vi "Get Motor Temperature Config.vi"(7 "timeout (1s)":dbl=1.0 min=0.0, 8 "error in (no error)":errorcluster, 11 "SDO object in":refnum<k20>) -> (0 "error out":errorcluster, 1 "completion codes":u32[](array[numeric]), 3 "SDO object out":refnum<k20>, 4 "Motor Temperature Config":T1)   [LabVIEW 2016]
uses:
  <vilib>/CANopenLib/CANOPEN.llb/CANopen SDO Read [U8].vi
  <vilib>/CANopenLib/CANOPEN.llb/CANopen SDO Read [I16].vi
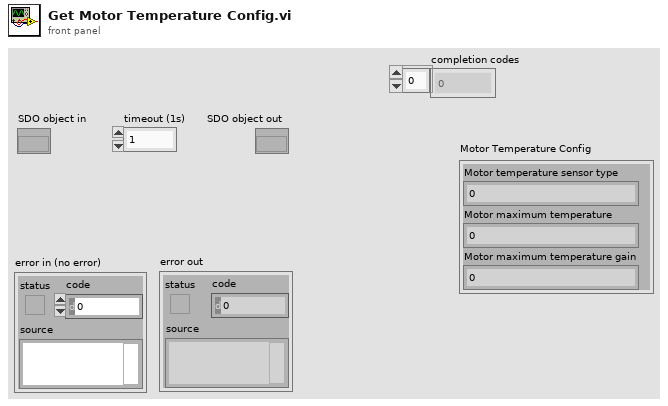
[diagram p1: front panel]
types:
  T1 = cluster{"Motor temperature sensor type":u8, "Motor maximum temperature":u8, "Motor maximum temperature gain":i16}
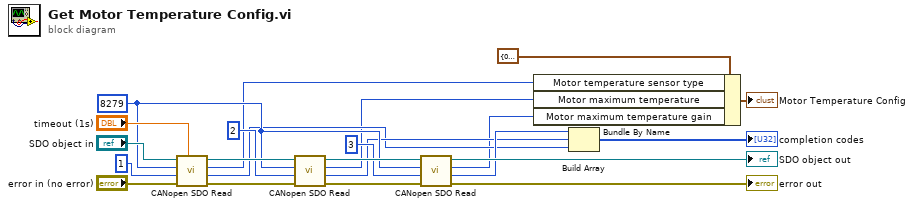
[diagram p0: block diagram]
diagram:
  w10 = u16 8279 ("object index")
  n1 = call-poly <vilib>:"CANopen SDO Read.vi"("timeout (1s)"="timeout (1s)", "error in (no error)"="error in (no error)", "object sub-index (0)"=u8 1, "object index"=w10, "SDO object in"="SDO object in") -> ("error out"=w19:errorcluster, "completion code"=w7:u32, "U8 data"=w4:u8, "SDO object out"=w18:refnum<k20>)  [unwired: 3 in]
  n2 = call-poly <vilib>:"CANopen SDO Read.vi"("error in (no error)"=w19, "object sub-index (0)"=u8 2, "object index"=w10, "SDO object in"=w18) -> ("error out"=w16:errorcluster, "completion code"=w8:u32, "U8 data"=w3:u8, "SDO object out"=w17:refnum<k20>)  [unwired: 4 in]
  n3 = call-poly <vilib>:"CANopen SDO Read.vi"("error in (no error)"=w16, "object sub-index (0)"=u8 3, "object index"=w10, "SDO object in"=w17) -> ("error out"=→"error out":errorcluster, "completion code"=w9:u32, "I16 data"=w2:i16, "SDO object out"=→"SDO object out":refnum<k20>)  [unwired: 4 in]
  n4 = Bundle By Name(cluster=T1 {"Motor temperature sensor type"=0, "Motor maximum temperature"=0, "Motor maximum temperature gain"=0} ("Motor Temperature Config"), "Motor temperature sensor type"=w4, "Motor maximum temperature"=w3, "Motor maximum temperature gain"=w2) -> (→"Motor Temperature Config":T1)
  n5 = Build Array(w9, w8, w7) -> (→"completion codes":u32[])
